vi "Task ID.vi"(8 "error in (no error)":errorcluster, 11 "ChartGuiTask in":refnum<class "ChartGuiTask.lvclass">) -> (0 "error out":errorcluster, 2 "Task ID":string, 3 "ChartGuiTask out":refnum<class "ChartGuiTask.lvclass">)   [LabVIEW 2020, in "VolatusDemo.lvlib" / "ChartGuiTask.lvclass"]
uses:
  ChartGuiTask.lvclass
  ChartGuiTask.lvclass/ChartGuiTask.ctl
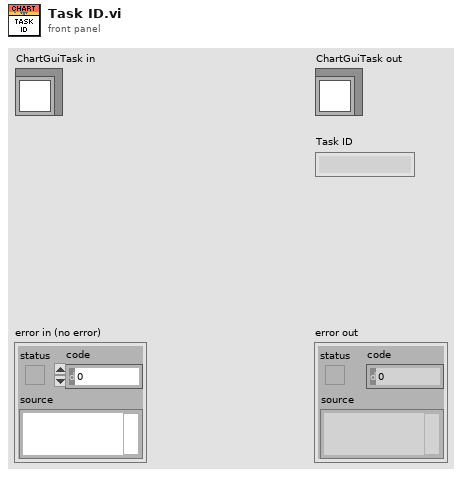
[diagram p1: front panel]
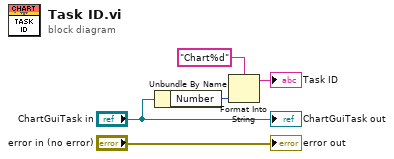
[diagram p0: block diagram]
diagram:
  n1 = Unbundle By Name("ChartGuiTask in") -> ("Number"=w2:i32)
  n2 = Format Into String(format string="Chart%d", w2) -> (resulting string=→"Task ID":string)  [unwired: 2 in, 1 out]
  "error out" <- "error in (no error)"
  "ChartGuiTask out" <- "ChartGuiTask in"
